vi "FindProjectPath.vi"(8 "error in (no error)":errorcluster, 10 "Library Name":string, 11 "Build Specs Folder Path":path) -> (0 "error out":errorcluster, 2 "Found?":bool, 3 "Project Path":path)   [LabVIEW 2023, in "Reusables.lvlib"]
uses:
  Reusables.lvlib
  <userlib>/_OpenG.lib/file/file.llb/openg_file.lvlib
  <vilib>/SLL Toolkit/SLL String/SLL String.lvlib
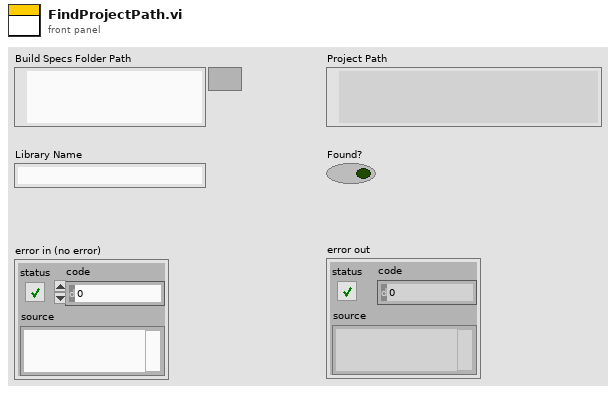
[diagram p1: front panel]
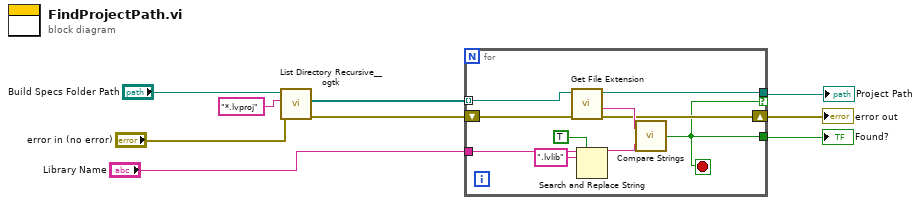
[diagram p0: block diagram]
diagram:
  n1 = call <userlib>:"List Directory Recursive__ogtk.vi"("error in (no error)"="error in (no error)", "pattern"="*.lvproj", "Path"="Build Specs Folder Path") -> ("error out"=w6:errorcluster, "file paths"=w4:path[])  [unwired: 5 in, 2 out]
  n2 = for {
    tunnel: w4 -> [w18] mode=indexing
    tunnel: "Library Name" -> [w17]
    shift-right: [w12] -> w1
    shift-left: w6 -> [w19]
    tunnel: [w11] -> w8 if=w10
    tunnel: [w10] -> w7
    stop <- w10 stop-if-true
    n3 = call <vilib>:"Get File Extension.vi"("error in (no error)"=w19, "file"=w18) -> ("error out"=w12:errorcluster, "filename without extension"=w14:string, "dup file"=w11:path)  [unwired: 5 in, 2 out]
    n4 = Search and Replace String(replace all?=TRUE ("replace all? (F)"), input string=w17, search string=".lvlib") -> (result string=w13:string)  [unwired: 5 in, 3 out]
    n5 = call <vilib>:"Compare Strings.vi"("y"=w13, "x"=w14) -> ("Equal?"=w10:bool)
  }
  "Project Path" <- w8
  "Found?" <- w7
  "error out" <- w1
